vi "Get Matrix - stdout.vi"(7 "is string?":bool, 8 "error in (no error)":errorcluster, 9 "octave sizes":i32[](array[numeric]), 10 "variable name":string, 11 "GOLPI ref. in":T1={"pipe handle"={"lv_proc.dll file path"=path "", "process instance handle"=[], "debug mode"=FALSE, "debug data"=[]}, "fast read timeout [ms]"=500, "fast read settle time [ms]"=10, "fast read to multiple [ms]"=1, "max elements per input line"=100, "slow read timeout [ms]"=5000, "stdin double format specifier"="%_16e", "max elements per stdout output column"=100}) -> (0 "error out":errorcluster, 2 "array":string[][](array[string]), 3 "GOLPI ref. out":T1={"pipe handle"={"lv_proc.dll file path"=path "", "process instance handle"=[], "debug mode"=FALSE, "debug data"=[]}, "fast read timeout [ms]"=500, "fast read settle time [ms]"=10, "fast read to multiple [ms]"=1, "max elements per input line"=100, "slow read timeout [ms]"=5000, "stdin double format specifier"="%_16e", "max elements per stdout output column"=100})   [LabVIEW 2013, in "GOLPI library.lvlib"]
doc: "Reads GNU Octave variable by means of stdout. The variable is in the form of the string, the conversion to doubles or complex must be done after. One has to select whether the variable is string."
uses:
  GOLPI library.lvlib
  Public/GOLPI reference Type Def.ctl
  LV Process source distribution/Pipe Handle.ctl
  Type Definitions/Custom Error Codes Enum Type Def.vi
  LV Process source distribution/LV Process library.lvlib
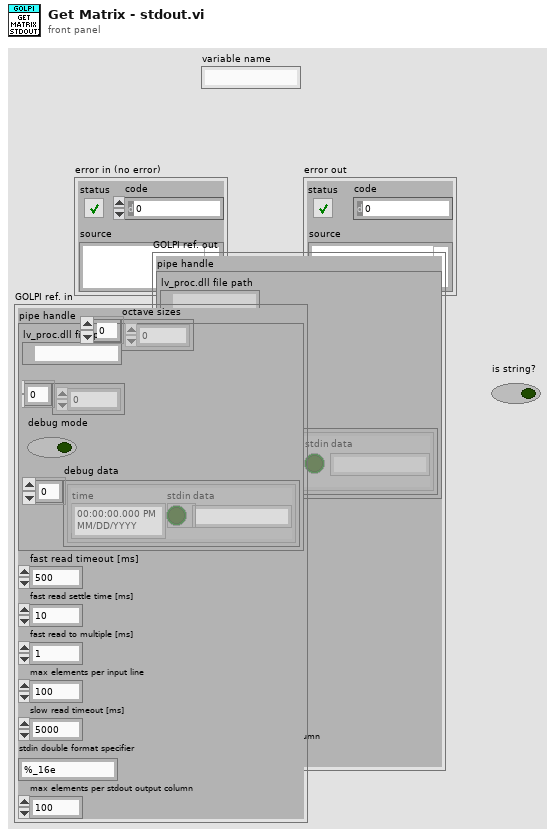
[diagram p1: front panel]
types:
  T1 = typedef "GOLPI library.lvlib/GOLPI reference Type Def.ctl" = cluster{"pipe handle":T2, "fast read timeout [ms]":u32, "fast read settle time [ms]":u32, "fast read to multiple [ms]":u32, "max elements per input line":u32, "slow read timeout [ms]":u32, "stdin double format specifier":string, "max elements per stdout output column":u32}
  T2 = typedef "LV Process library.lvlib/Pipe Handle.ctl" = cluster{"lv_proc.dll file path":path, "process instance handle":u32[], "debug mode":bool, "debug data":cluster{"time":timestamp, "stdin":bool, "data":string}[]}
  T3 = typedef "GOLPI library.lvlib/Custom Error Codes Enum Type Def.vi" = enum16{"no error", "00 working directory PAR1 missing", "01 octave binary PAR1 missing", "02 octave report error PAR1", "03 empty output last cmd PAR1", "04 missing temporary file PAR1", "05 pwd PAR 1 not exist", "10 var PAR1 not string, vect", "11 var PAR1 not num, scal, ~compl", "12 var PAR1 not num, scal, compl", "13 var PAR1 not num, vect, ~compl", "14 var PAR1 not num, vect, compl", "15 var PAR1 not num, mat, ~compl", "16 var PAR1 not num, mat, ~compl", "30 WARNING read timeout", "99 not finished"}
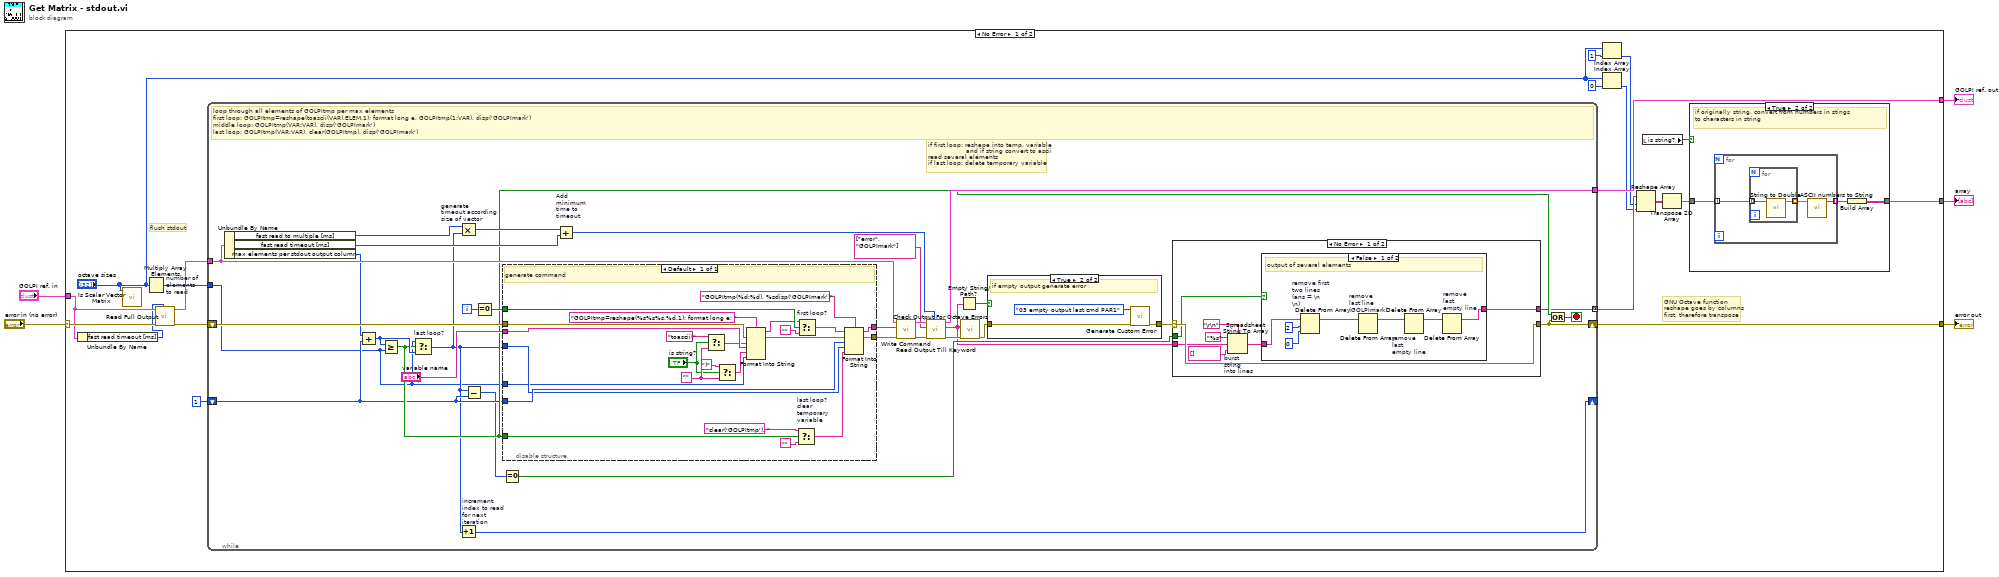
[diagram p0: block diagram]
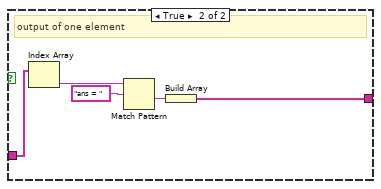
[diagram p4: hidden frame]
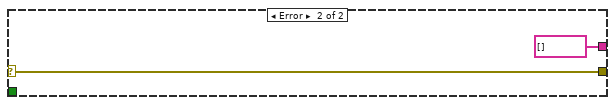
[diagram p5: hidden frame]
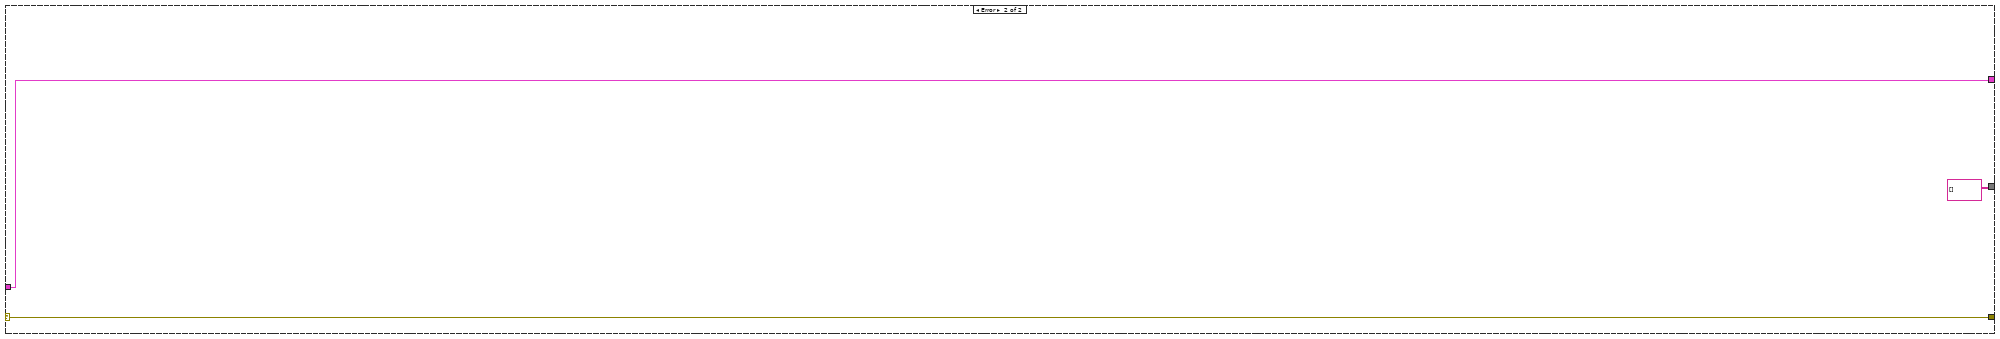
[diagram p6: hidden frame]
diagram:
  n1 = case shown="No Error" "error in (no error)" {
    selector: "error in (no error)" -> [w20 w118]
    tunnel: "GOLPI ref. in" -> [w7 w117]
    tunnel: [w18 w118] -> w5
    tunnel: [w24 w117] -> w2
    tunnel: [w8 string[][] []] -> w1
    frame No Error {
      # "GNU Octave function\nreshape goes by columns\nfirst, therefore transpose"
      # "flush stdout"
      # "if octave not reported error"
      n2 = Unbundle By Name(w7) -> ("fast read timeout [ms]"=w6:u32)
      n3 = call "Is Scalar Vector Matrix.vi"("octave sizes"="octave sizes") -> ()  [unwired: 5 in, 6 out]
      n4 = Multiply Array Elements "number of\nelements\nto read"(1:"octave sizes") -> (0:w22:i32)
      n5 = call "Read Full Output.vi"("timeout [ms]"=w6, "error in"=w20, "GOLPI ref. in"=w7) -> ("error out"=w21:errorcluster, "GOLPI ref. out"=w19:T1)  [unwired: 5 in, 2 out]
      n6 = while {
        tunnel: w19 -> [w54]
        tunnel: [w57] -> w24
        shift-right: [w46] -> w18
        shift-left: w21 -> [w50]
        tunnel: w22 -> [w36]
        shift-right: [w55] -> _
        shift-left: u32 1 ("input 1") -> [w41]
        tunnel: [w38] -> w17 mode=concatenating
        i -> [w52]
        stop <- w47 stop-if-true
        # "if first loop: reshape into temp. variable\n                   and if string convert to ascii\nread several elements\nif last loop: delete temporary variable"
        # "loop through all elements of GOLPItmp per max elements\nfirst loop: GOLPItmp=reshape(toascii(VAR),ELEM,1); format long e, GOLPItmp(1:VAR), disp('GOLPImark')\nmiddle loop: GOLPItmp(VAR:VAR), disp('GOLPImark')\nlast loop: GOLPItmp(VAR:VAR), clear(GOLPItmp), disp('GOLPImark')"
        n7 = Unbundle By Name(w54) -> ("fast read to multiple [ms]"=w58:u32, "fast read timeout [ms]"=w59:u32, "max elements per stdout output column"=w34:u32)
        n8 = Add(x=w34, y=w41) -> (x+y=w56:u32)
        n9 = Greater Or Equal?(x=w56, y=w36) -> (x >= y?=w48:bool)
        n10 = Select "last loop?"(t=w36, s=w48, f=w56) -> (s? t:f=w37:u32)
        n11 = Multiply "generate\ntimeout according\nsize of vector"(x=w58, y=w37) -> (x*y=w62:u32)
        n12 = Increment "increment\nindex to read\nfor next\niteration"(x=w37) -> (x+1=w55:u32)
        n13 = Subtract(x=w37, y=w41) -> (x-y=w35:u32)
        n14 = Equal To 0?(x=w52) -> (x = 0?=w51:bool)
        n15 = disable-structure shown="Default" {
          disable-tunnel: [w88] -> w60
          disable-tunnel: [w87] -> w53
          disable-tunnel: w51 -> [w86]
          disable-tunnel: w50 -> [w81]
          disable-tunnel: "variable name" -> [w77]
          disable-tunnel: w48 -> [w71]
          disable-tunnel: w41 -> [w70]
          disable-tunnel: w37 -> [w69]
          disable-tunnel: w36 -> [w66]
          frame Enabled {
            w74 = ""
            # "generate command"
            n16 = Select(t="toascii(" ("format string"), s="is string?", f=w74) -> (s? t:f=w75:string)
            n17 = Select(t=")", s="is string?", f=w74) -> (s? t:f=w72:string)
            n18 = Format Into String(format string="GOLPItmp=reshape(%s%s%s,%d,1); format long e; ", error in=w81, w75, w77, w72, w66) -> (resulting string=w79:string, error out=w82:errorcluster)  [unwired: 1 in]
            n19 = Select "last loop?\nclear\ntemporary\nvariable"(t="clear('GOLPItmp'), " ("format string"), s=w71, f="") -> (s? t:f=w83:string)
            n20 = Select "first loop?"(t=w79, s=w86, f="") -> (s? t:f=w78:string)
            n21 = Format Into String(format string="GOLPItmp(%d:%d), %sdisp('GOLPImark')", initial string=w78, error in=w82, w70, w69, w83) -> (resulting string=w88:string, error out=w87:errorcluster)
          }
        }
        n22 = Equal To 0?(x=w35) -> (x = 0?=w40:bool)
        n23 = Add "Add\nminimum\ntime to\ntimeout"(x=w62, y=w59) -> (x+y=w61:u32)
        n24 = call "Write Command.vi"("error in"=w53, "command"=w60, "GOLPI ref. in"=w54) -> ("error out"=w63:errorcluster, "GOLPI ref. out"=w65:T1)  [unwired: 7 in]
        n25 = call "Read Output Till Keyword.vi"("timeout [ms]"=w61, "error in"=w63, "keywords"=string[] ["error", "GOLPImark"], "GOLPI ref. in"=w65) -> ("error out"=w44:errorcluster, "read buffer"=w39:string, "GOLPI ref. out"=w57:T1)  [unwired: 4 in, 1 out]
        n26 = Empty String/Path?(string/path=w39) -> (empty?=w45:bool)
        n27 = call "Check Output For Octave Errors.vi"("error in"=w44, "read buffer"=w39) -> ("error out"=w43:errorcluster)  [unwired: 9 in]
        n28 = case shown="True" w45 {
          tunnel: w43 -> [w90 w92]
          tunnel: [w90 w91] -> w42
          frame False {
          }
          frame True {
            # "if empty output generate error"
            n29 = call "Generate Custom Error.vi"("error in"=w92, "GOLPI error"=Custom_Error_Codes_Enum_Type_Def.vi."03 empty output last cmd PAR1" ("Enum")) -> ("error out"=w91:errorcluster)  [unwired: 9 in]
          }
        }
        n30 = case shown="No Error" w42 {
          selector: w42 -> [w101 w115]
          tunnel: [w101 w115] -> w46
          tunnel: w40 -> [w100 _]
          tunnel: w39 -> [w95 _]
          tunnel: [w99 string[] []] -> w38
          frame No Error {
            n31 = Spreadsheet String To Array "burst\nstring\ninto lines"(delimiter (Tab)="\r\n", format string="%s", spreadsheet string=w95, array type (2D Dbl)=string[] []) -> (array=w94:string[])
            n32 = case shown="False" w100 {
              tunnel: [w104 w111] -> w99
              tunnel: w94 -> [w102 w110]
              frame False {
                # "output of several elements"
                n33 = Delete From Array "remove first\ntwo lines\n(ans = \\n\n\\n)"(array=w102, length=2, index=0) -> (array with subset deleted=w106:string[])  [unwired: 1 out]
                n34 = Delete From Array "remove\nlast line\n(GOLPImark)"(array=w106) -> (array with subset deleted=w105:string[])  [unwired: 2 in, 1 out]
                n35 = Delete From Array "remove\nlast\nempty line"(array=w105) -> (array with subset deleted=w103:string[])  [unwired: 2 in, 1 out]
                n36 = Delete From Array "remove\nlast\nempty line"(array=w103) -> (array with subset deleted=w104:string[])  [unwired: 2 in, 1 out]
              }
              frame True {
                # "output of one element"
                n37 = Index Array(array=w110) -> (element=w109:string)  [unwired: 1 in]
                n38 = Match Pattern(string=w109, regular expression="ans = ") -> (after substring=w112:string)  [unwired: 1 in, 3 out]
                n39 = Build Array(w112) -> (w111:string[])
              }
            }
          }
          frame Error {
          }
        }
        n40 = Or(x=w48, y=w46) -> (x .or. y?=w47:bool)
      }
      n41 = Index Array(array="octave sizes", index=1) -> (element=w13:i32)
      n42 = Index Array(array="octave sizes", index=0) -> (element=w12:i32)
      n43 = Reshape Array(w17, w13, w12) -> (w11:string[][])
      n44 = local read "is string?"() -> (w10:bool)
      n45 = Transpose 2D Array(2D array=w11) -> (transposed array=w9:string[][])
      n46 = case shown="True" w10 {
        tunnel: [w25 w27] -> w8
        tunnel: w9 -> [w25 w26]
        frame False {
        }
        frame True {
          # "if originally string, convert from numbers in stings\nto characters in string"
          n47 = for {
            tunnel: [w31] -> w28 mode=indexing
            tunnel: w26 -> [w29] mode=indexing
            n48 = for {
              tunnel: [w33] -> w30 mode=indexing
              tunnel: w29 -> [w32] mode=indexing
              n49 = call "String to Double.vi"("string"=w32) -> ("number"=w33:dbl)  [unwired: 10 in]
            }
            n50 = call "ASCII numbers to String.vi"("ascii numbers"=w30) -> ("string"=w31:string)  [unwired: 10 in]
          }
          n51 = Build Array(w28) -> (w27:string[][])
        }
      }
    }
    frame Error {
    }
  }
  "error out" <- w5
  "GOLPI ref. out" <- w2
  "array" <- w1
